vi "DataValueFromString.vi"(4 "label":bool, 5 "Type":variant, 8 "value":string, 9 "module namespace":string="lvDT.") -> (3 "value":string)   [LabVIEW 2014, in "Python Functions.lvlib"]
uses:
  Parsing/Python Functions.lvlib
  <vilib>/Utility/VariantDataType/Type.ctl
  <vilib>/Utility/VariantDataType/VariantType.lvlib
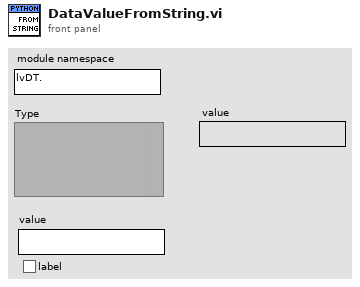
[diagram p1: front panel]
types:
  T1 = typedef "VariantType.lvlib/Type.ctl" = enum8{"Invalid Type", "Void", "I8", "I16", "I32", "I64", "U8", "U16", "U32", "U64", "Single Float", "Double Float", "Extended Float", "Single Complex", "Double Complex", "Extended Complex", "Enum U8", "Enum U16", "Enum U32", "Enum U64", "Single Float With Unit", "Double Float With Unit", "Extended Float With Unit", "Single Complex with Unit", "Double Complex with Unit", "Extended Complex with Unit", "Boolean", "String", "Path", "Picture", "Tag", "Array", "Cluster", "Variant", "LV Variant", "Waveform", "Timestamp", "Digital Waveform", "Digital Data", "ExpressData", "Refnum", "External Data", "VI", "Poly VI", "LabVIEW Class Instance", "Fixed Point"}
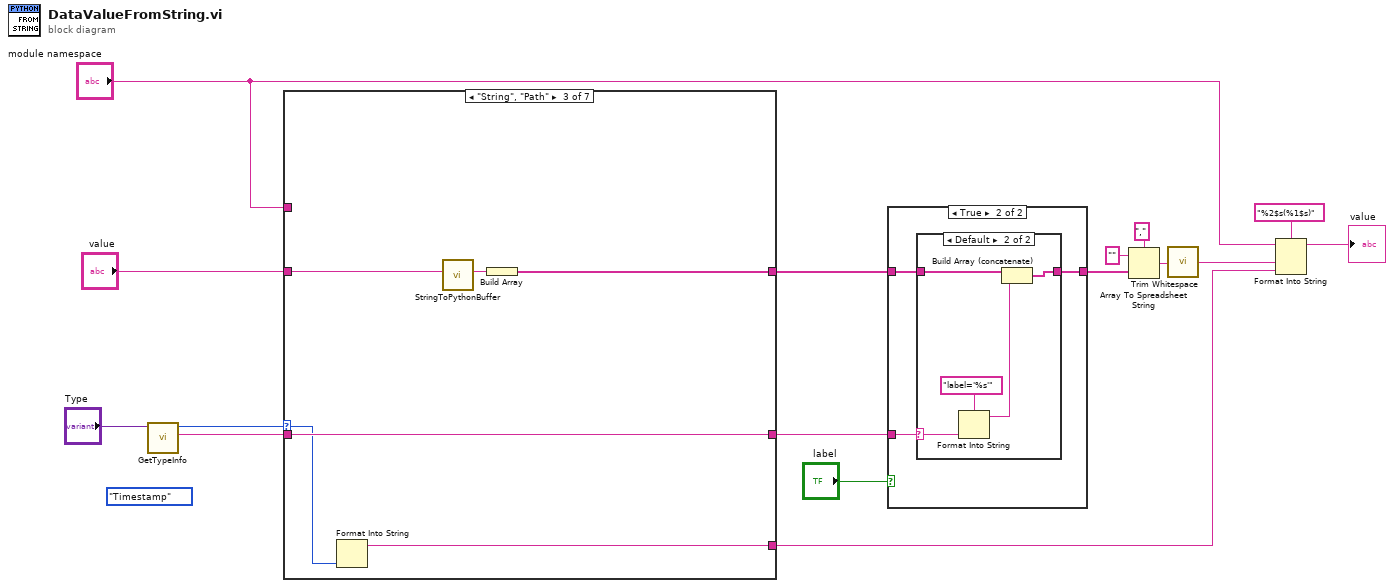
[diagram p0: block diagram]
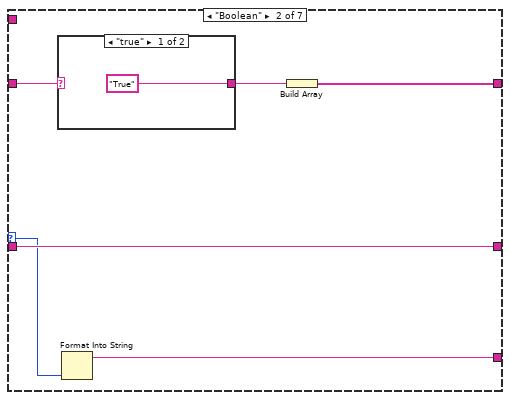
[diagram p5: hidden frame]
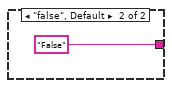
[diagram p6: hidden frame]
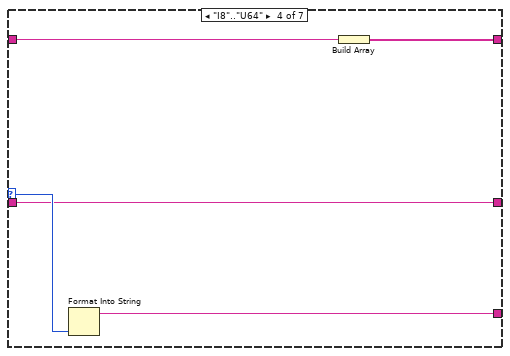
[diagram p7: hidden frame]
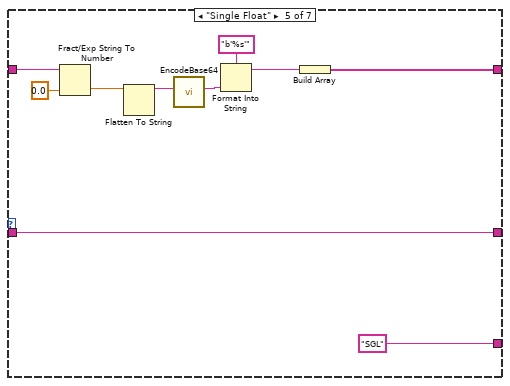
[diagram p8: hidden frame]
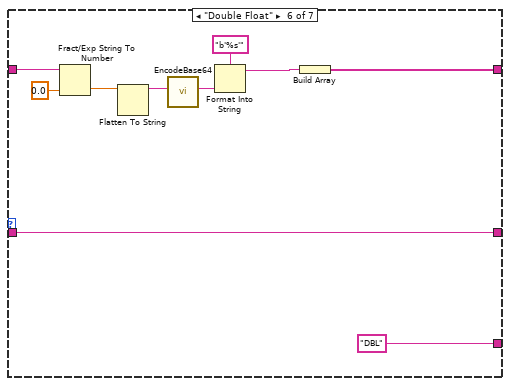
[diagram p9: hidden frame]
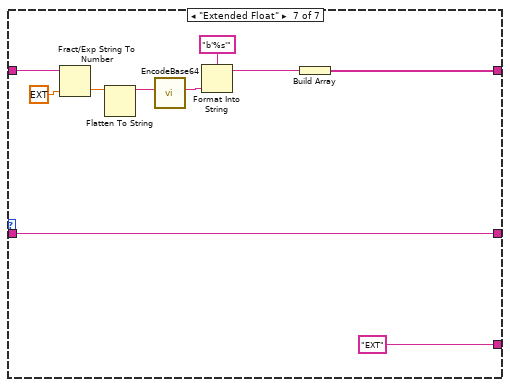
[diagram p10: hidden frame]
diagram:
  (unwired) Type."Timestamp" ("Type Enum")
  n1 = call <vilib>:"GetTypeInfo.vi"("Variant"="Type") -> ("Name"=w15:string, "Type Enum"=w16:T1)  [unwired: 6 in, 3 out]
  n2 = case shown="\"String\", \"Path\"" w16 {
    selector: w16 -> [_ w21 w29 w35 _ _ _]
    tunnel: "module namespace" -> [_ _ _ _ _ _ _]
    tunnel: [_ w20 w28 w33 w44 w54 w64] -> w3
    tunnel: w15 -> [w17 w23 w31 w34 w45 w55 w65]
    tunnel: [w17 w23 w31 w34 w45 w55 w65] -> w14
    tunnel: [_ w22 w30 w36 "SGL" "DBL" "EXT"] -> w7
    tunnel: "value" -> [_ w19 w26 w32 w40 w50 w60]
    frame Default {
    }
    frame "Boolean" {
      n3 = case shown="\"true\"" w19 {
        tunnel: ["True" "False"] -> w18
        frame "true" {
        }
        frame "false", Default {
        }
      }
      n4 = Format Into String(w21) -> (resulting string=w22:string)  [unwired: 3 in, 1 out]
      n5 = Build Array(w18) -> (w20:string[])
    }
    frame "String", "Path" {
      n6 = Format Into String(w29) -> (resulting string=w30:string)  [unwired: 3 in, 1 out]
      n7 = call "StringToPythonBuffer.vi"("string"=w26) -> ("python string"=w27:string)  [unwired: 8 in]
      n8 = Build Array(w27) -> (w28:string[])
    }
    frame "I8".."U64" {
      n9 = Format Into String(w35) -> (resulting string=w36:string)  [unwired: 3 in, 1 out]
      n10 = Build Array(w32) -> (w33:string[])
    }
    frame "Single Float" {
      n11 = Fract/Exp String To Number(string=w40, default (0 dbl)=sgl 0.0) -> (number=w37:sgl)  [unwired: 2 in, 1 out]
      n12 = Flatten To String(anything=w37) -> (data string=w38:string)  [unwired: 3 in, 2 out]
      n13 = call "EncodeBase64.vi"("string"=w38) -> ("base64 string"=w42:string)  [unwired: 10 in]
      n14 = Format Into String(format string="b'%s'", w42) -> (resulting string=w41:string)  [unwired: 2 in, 1 out]
      n15 = Build Array(w41) -> (w44:string[])
    }
    frame "Double Float" {
      n16 = Fract/Exp String To Number(string=w50, default (0 dbl)=0.0) -> (number=w47:dbl)  [unwired: 2 in, 1 out]
      n17 = Flatten To String(anything=w47) -> (data string=w48:string)  [unwired: 3 in, 2 out]
      n18 = call "EncodeBase64.vi"("string"=w48) -> ("base64 string"=w52:string)  [unwired: 10 in]
      n19 = Format Into String(format string="b'%s'", w52) -> (resulting string=w51:string)  [unwired: 2 in, 1 out]
      n20 = Build Array(w51) -> (w54:string[])
    }
    frame "Extended Float" {
      n21 = Fract/Exp String To Number(string=w60, default (0 dbl)=ext 0.0) -> (number=w57:ext)  [unwired: 2 in, 1 out]
      n22 = Flatten To String(anything=w57) -> (data string=w58:string)  [unwired: 3 in, 2 out]
      n23 = call "EncodeBase64.vi"("string"=w58) -> ("base64 string"=w62:string)  [unwired: 10 in]
      n24 = Format Into String(format string="b'%s'", w62) -> (resulting string=w61:string)  [unwired: 2 in, 1 out]
      n25 = Build Array(w61) -> (w64:string[])
    }
  }
  n26 = case shown="True" "label" {
    tunnel: w14 -> [_ w68]
    tunnel: w3 -> [w67 w70]
    tunnel: [w67 w69] -> w12
    frame False {
    }
    frame True {
      n27 = case shown="Default" w68 {
        selector: w68 -> [_ w72]
        tunnel: w70 -> [w71 w76]
        tunnel: [w71 w75] -> w69
        frame "" {
        }
        frame Default {
          n28 = Format Into String(format string="label='%s'", w72) -> (resulting string=w73:string)  [unwired: 2 in, 1 out]
          n29 = Build Array (concatenate)(w76, w73) -> (w75:string[])
        }
      }
    }
  }
  n30 = Array To Spreadsheet String(delimiter (Tab)=",", array=w12, 3:"" ("format string")) -> (spreadsheet string=w10:string)
  n31 = call <vilib>:"Trim Whitespace.vi"("string"=w10) -> ("trimmed string"=w8:string)  [unwired: 1 in]
  n32 = Format Into String(format string="%2$s(%1$s)", initial string="module namespace", w8, w7) -> (resulting string=→"value":string)  [unwired: 1 in, 1 out]
